vi "Enqueue Write Multi D.vi"(7 "D Array":i16[](array[numeric]), 8 "Error In":errorcluster, 9 "Length (U16)":u16, 10 "Position (U32)":u32, 11 "Name":string) -> (0 "Error Out":errorcluster)   [LabVIEW 2019, in "FX5U SLMP Binary.lvlib"]
uses:
  FX5U SLMP Binary.lvlib
  Queue/Queue.lvlib
  Error Notifier/Error Notifier.lvlib
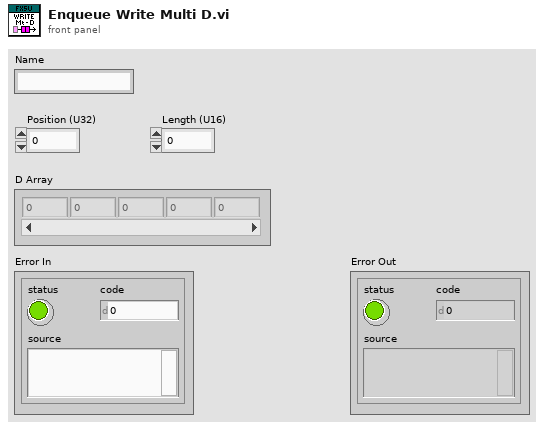
[diagram p1: front panel]
types:
  T1 = cluster{"Position (U32)":u32, "Length (U16)":u16, "D Array":i16[]}
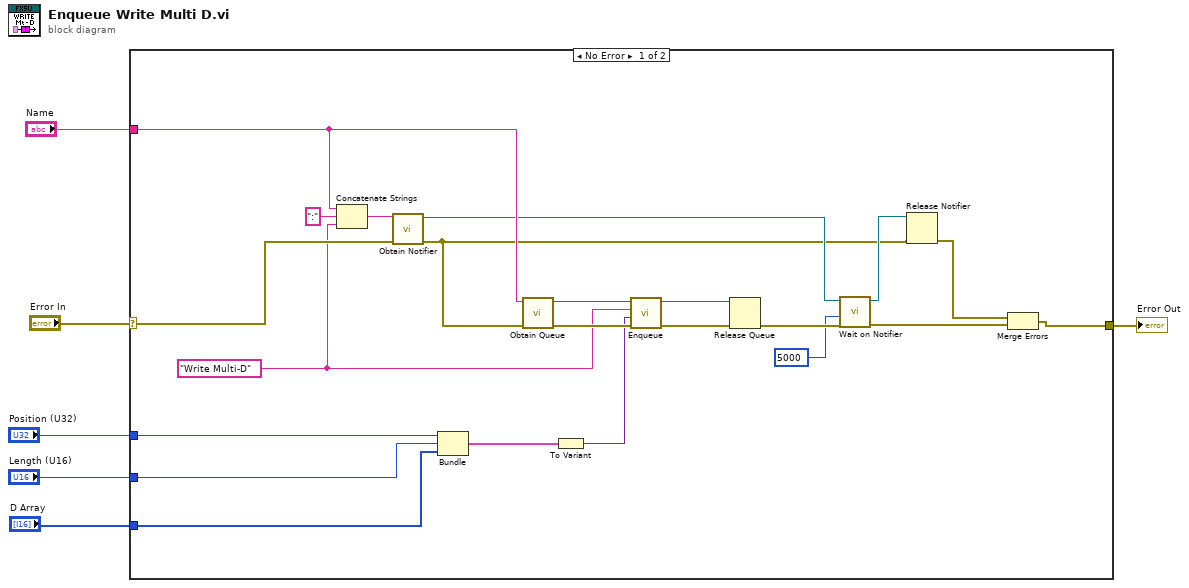
[diagram p0: block diagram]
diagram:
  n1 = case shown="No Error" "Error In" {
    selector: "Error In" -> [w28 w29]
    tunnel: [w13 w29] -> w5
    tunnel: "Name" -> [w26 _]
    tunnel: "Position (U32)" -> [w11 _]
    tunnel: "D Array" -> [w7 _]
    tunnel: "Length (U16)" -> [w8 _]
    frame No Error {
      w23 = "Write Multi-D" ("Message")
      n2 = Concatenate Strings(w26, ":" ("string"), w23) -> (w25:string)
      n3 = call "Obtain Notifier.vi"("Error In"=w28, "Name"=w25) -> ("Error Out"=w12:errorcluster, "notifier out"=w18:refnum<notifier>)  [unwired: 8 in]
      n4 = Bundle("Position (U32)"=w11, "Length (U16)"=w8, "D Array"=w7) -> (w10:T1)  [unwired: 1 in]
      n5 = call "Obtain Queue.vi"("Error In"=w12, "Name"=w26) -> ("Error Out"=w27:errorcluster, "queue out"=w21:refnum<queue>)  [unwired: 8 in]
      n6 = To Variant(anything=w10) -> (Variant=w9:variant)
      n7 = call "Enqueue.vi"("Error In"=w27, "Data"=w9, "Message"=w23, "queue in"=w21) -> ("Error Out"=w22:errorcluster, "queue out"=w20:refnum<queue>)  [unwired: 6 in]
      n8 = Release Queue(queue=w20, error in (no error)=w22) -> (error out=w19:errorcluster)  [unwired: 1 in, 2 out]
      n9 = call "Wait on Notifier.vi"("Error In"=w19, "timeout in ms (-1)"=5000, "notifier in"=w18) -> ("Error Out"=w14:errorcluster, "notifier out"=w16:refnum<notifier>)  [unwired: 7 in]
      n10 = Release Notifier(notifier=w16, error in (no error)=w12) -> (error out=w15:errorcluster)  [unwired: 1 in, 2 out]
      n11 = Merge Errors(w15, w14) -> (w13:errorcluster)
    }
    frame Error {
    }
  }
  "Error Out" <- w5
